vi "TDMS_CREATE.vi"() -> ()   [LabVIEW 2021]
uses:
  <vilib>/Utility/TDMS File Viewer/NI_TDMS File Viewer.lvlib
panel:
  in  "File Path":path
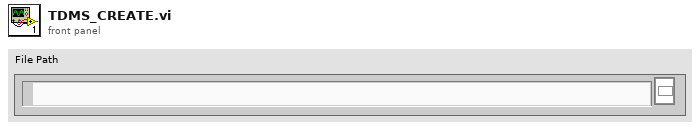
[diagram p1: front panel]
types:
  T1 = enum16{"open", "open or create", "create or replace", "create", "open (read-only)"}
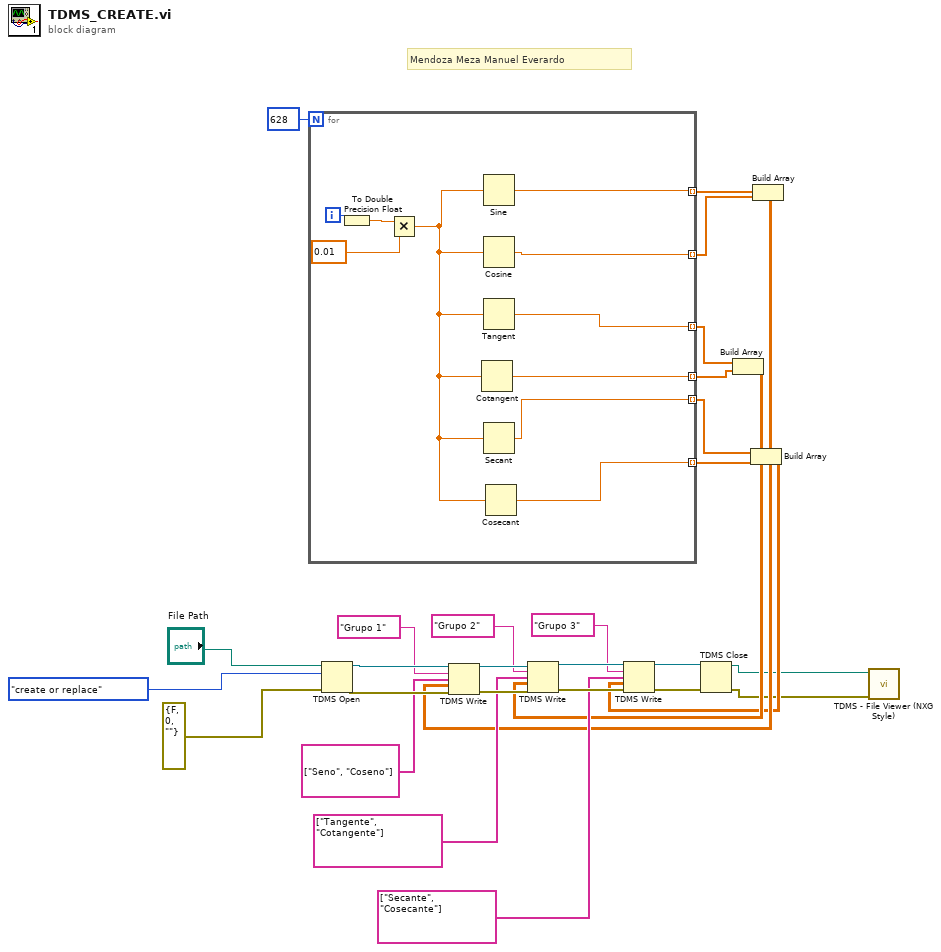
[diagram p0: block diagram]
diagram:
  # "Mendoza Meza Manuel Everardo"
  n1 = for {
    N: 628 -> [_]
    tunnel: [w36] -> w14 mode=indexing
    tunnel: [w35] -> w13 mode=indexing
    tunnel: [w34] -> w11 mode=indexing
    tunnel: [w33] -> w8 mode=indexing
    tunnel: [w32] -> w7 mode=indexing
    tunnel: [w31] -> w9 mode=indexing
    i -> [w38]
    n2 = To Double Precision Float(number=w38) -> (double precision float=w37:dbl)
    n3 = Multiply(x=w37, y=0.01) -> (x*y=w30:dbl)
    n4 = Cotangent(1:w30) -> (0:w31:dbl)
    n5 = Sine(x=w30) -> (sin(x)=w36:dbl)
    n6 = Cosine(x=w30) -> (cos(x)=w35:dbl)
    n7 = Tangent(1:w30) -> (0:w34:dbl)
    n8 = Secant(1:w30) -> (0:w33:dbl)
    n9 = Cosecant(1:w30) -> (0:w32:dbl)
  }
  n10 = TDMS Open(8:errorcluster {"status"=FALSE, "code"=0, "source"=""} ("error in (no error)"), 10:T1."create or replace" ("operation (0:open)"), 11:"File Path") -> (0:w25:errorcluster, 3:w26:refnum<k34>)  [unwired: 4 in]
  n11 = Build Array(w11, w9) -> (w10:dbl[][])
  n12 = Build Array(w8, w7) -> (w6:dbl[][])
  n13 = Build Array(w14, w13) -> (w12:dbl[][])
  n14 = TDMS Write(0:w26, 5:"Grupo 1" ("group name in (Untitled)"), 7:string[] ["Seno", "Coseno"] ("channel name(s) in (Untitled)"), 9:w12, 11:w25) -> (4:w24:refnum<k34>, 15:w23:errorcluster)  [unwired: 1 in, 2 out]
  n15 = TDMS Write(0:w24, 5:"Grupo 2" ("group name in (Untitled)"), 7:string[] ["Tangente", "Cotangente"] ("channel name(s) in (Untitled)"), 9:w10, 11:w23) -> (4:w21:refnum<k34>, 15:w22:errorcluster)  [unwired: 1 in, 2 out]
  n16 = TDMS Write(0:w21, 5:"Grupo 3" ("group name in (Untitled)"), 7:string[] ["Secante", "Cosecante"] ("channel name(s) in (Untitled)"), 9:w6, 11:w22) -> (4:w5:refnum<k34>, 15:w4:errorcluster)  [unwired: 1 in, 2 out]
  n17 = TDMS Close(8:w4, 11:w5) -> (0:w3:errorcluster, 3:w1:path)
  n18 = call <vilib>:"TDMS - File Viewer (NXG Style).vi"("error in"=w3, "file in"=w1) -> ()  [unwired: 8 in, 2 out]
